vi "saveSettings.vi"(8 "error in (no error)":errorcluster, 10 "Path":path, 11 "ICSettingsViewer in":refnum<class "ICSettingsViewer.lvclass">) -> (0 "error out":errorcluster, 3 "ICSettingsViewer out":refnum<class "ICSettingsViewer.lvclass">)   [LabVIEW 2011, in "Views.lvlib" / "Camera.lvlib" / "ICSettingsViewer.lvclass"]
uses:
  ICSettingsViewer.lvclass
  Tools/SettingsEventManager/SettingsEventsManager.lvclass
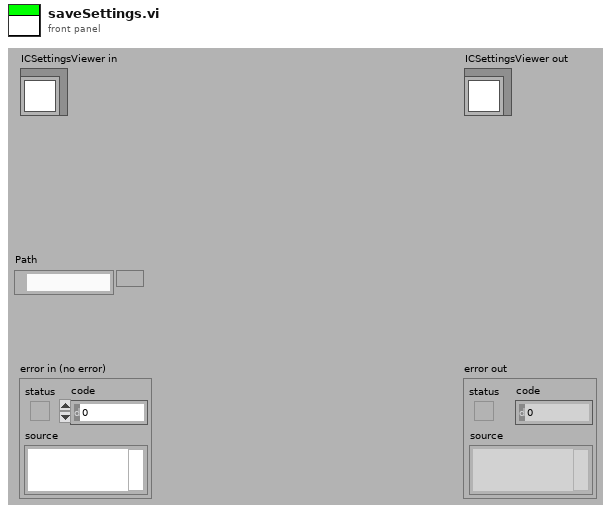
[diagram p1: front panel]
types:
  T1 = cluster{"settingsFrontEndEvents":cluster{"loadSettingsFromPath":refnum<user-event>, "lookUpElementEvent":refnum<user-event>, "saveSettings":refnum<user-event>, "loadSettings":refnum<user-event>, "close":refnum<user-event>, "replaceElement":refnum<user-event>, "findParentNodes":refnum<user-event>, "createNode":refnum<user-event>}, "settingBackEndEvents":cluster{"defaultSettingsPathRequest":refnum<user-event>, "searchResultEvent":refnum<user-event>, "settingsSaved":refnum<user-event>, "settingsLoaded":refnum<user-event>, "foundParentNode":refnum<user-event>}}
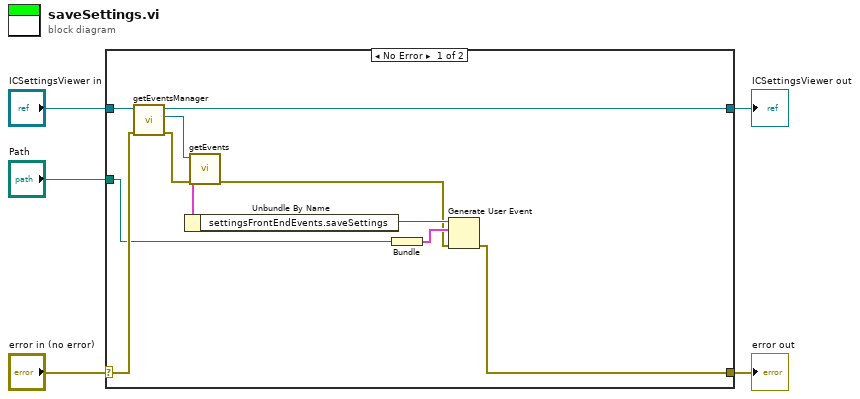
[diagram p0: block diagram]
diagram:
  n1 = case shown="No Error" "error in (no error)" {
    selector: "error in (no error)" -> [w13 w18]
    tunnel: [w7 w18] -> w4
    tunnel: [w6 w17] -> w2
    tunnel: "ICSettingsViewer in" -> [w14 w17]
    tunnel: "Path" -> [w10 _]
    frame No Error {
      n2 = call-dynamic "getEventsManager.vi"("error in (no error)"=w13, "SettingsViewer.lvclass in"=w14) -> ("error out"=w15:errorcluster, "Tools.lvlib:Settings.lvlib:SettingsEventsManager.lvclass"=w16:refnum<class "SettingsEventsManager.lvclass">, "SettingsViewer.lvclass out"=w6:refnum<class "ICSettingsViewer.lvclass">)  [unwired: 7 in]
      n3 = call-dynamic "getEvents.vi"("error in (no error)"=w15, "SettingsEventsManager in"=w16) -> ("error out"=w8:errorcluster, "settingsEvents"=w12:T1)  [unwired: 7 in, 1 out]
      n4 = Unbundle By Name(w12) -> ("settingsFrontEndEvents.saveSettings"=w11:refnum<user-event>)
      n5 = Bundle("Path"=w10) -> (w9:cluster{"Path":path})  [unwired: 1 in]
      n6 = Generate User Event(user event=w11, event data cluster=w9, error in=w8) -> (error out=w7:errorcluster)  [unwired: 1 out]
    }
    frame Error {
    }
  }
  "error out" <- w4
  "ICSettingsViewer out" <- w2
